vi "event_indicies.vi"(7 "wavelet array length":i32, 10 "Input Outlier indices":T1) -> (0 "t_c":cluster{"t_start_c":dbl[], "t_end_c":dbl[]}, 1 "t_b":cluster{"t_start_b":dbl[], "t_end_b":dbl[]}, 2 "t_a":cluster{"t_start_a":dbl[], "t_end_a":dbl[]})   [LabVIEW 2014]
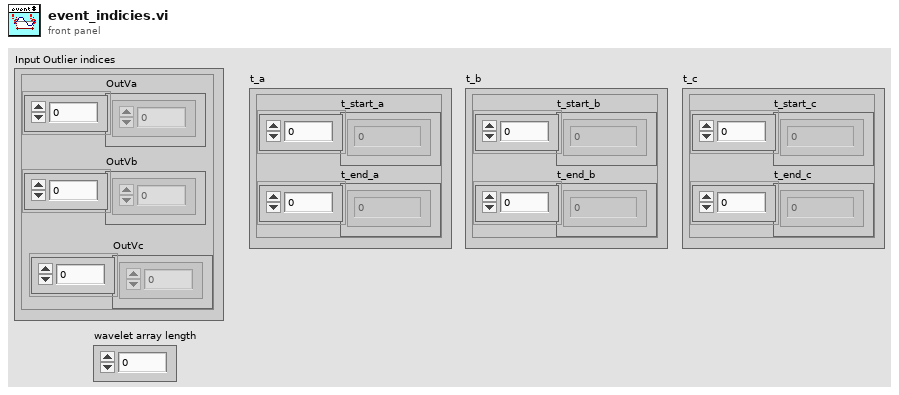
[diagram p1: front panel]
types:
  T1 = cluster{"OutVa":i32[], "OutVb":i32[], "OutVc":i32[]}
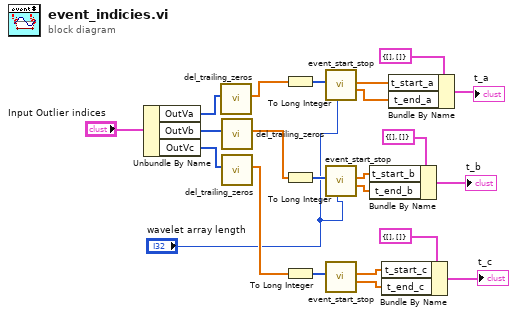
[diagram p0: block diagram]
diagram:
  n1 = Unbundle By Name("Input Outlier indices") -> ("OutVa"=w22:i32[], "OutVb"=w20:i32[], "OutVc"=w18:i32[])
  n2 = call "del_trailing_zeros.vi"("Array"=w22) -> ("Shortened array"=w21:dbl[])  [unwired: 10 in]
  n3 = call "del_trailing_zeros.vi"("Array"=w20) -> ("Shortened array"=w19:dbl[])  [unwired: 10 in]
  n4 = call "del_trailing_zeros.vi"("Array"=w18) -> ("Shortened array"=w17:dbl[])  [unwired: 10 in]
  n5 = To Long Integer(number=w21) -> (32bit integer=w16:i32[])
  n6 = To Long Integer(number=w19) -> (32bit integer=w15:i32[])
  n7 = To Long Integer(number=w17) -> (32bit integer=w14:i32[])
  n8 = call "event_start_stop.vi"("Wavelet Array Length"="wavelet array length", "Event Indices"=w16) -> ("Event End Time"=w11:dbl[], "Event Start Time"=w12:dbl[])  [unwired: 8 in]
  n9 = call "event_start_stop.vi"("Wavelet Array Length"="wavelet array length", "Event Indices"=w15) -> ("Event End Time"=w8:dbl[], "Event Start Time"=w9:dbl[])  [unwired: 8 in]
  n10 = call "event_start_stop.vi"("Event Indices"=w14) -> ("Event End Time"=w4:dbl[], "Event Start Time"=w5:dbl[])  [unwired: 9 in]
  n11 = Bundle By Name(cluster=cluster{"t_start_b":dbl[], "t_end_b":dbl[]} {"t_start_b"=[], "t_end_b"=[]} ("t_b"), "t_start_b"=w9, "t_end_b"=w8) -> (→"t_b":cluster{"t_start_b":dbl[], "t_end_b":dbl[]})
  n12 = Bundle By Name(cluster=cluster{"t_start_c":dbl[], "t_end_c":dbl[]} {"t_start_c"=[], "t_end_c"=[]} ("t_c"), "t_start_c"=w5, "t_end_c"=w4) -> (→"t_c":cluster{"t_start_c":dbl[], "t_end_c":dbl[]})
  n13 = Bundle By Name(cluster=cluster{"t_start_a":dbl[], "t_end_a":dbl[]} {"t_start_a"=[], "t_end_a"=[]} ("t_a"), "t_start_a"=w12, "t_end_a"=w11) -> (→"t_a":cluster{"t_start_a":dbl[], "t_end_a":dbl[]})
